vi "Make Graph.vi"(10 "SciData":dbl[][](array[numeric]), 11 "X-Data":dbl[](array[numeric])) -> (3 "All Counts 2":cluster{"X-Data":dbl[], "SciData":dbl[]}[](graph))   [LabVIEW 2025]
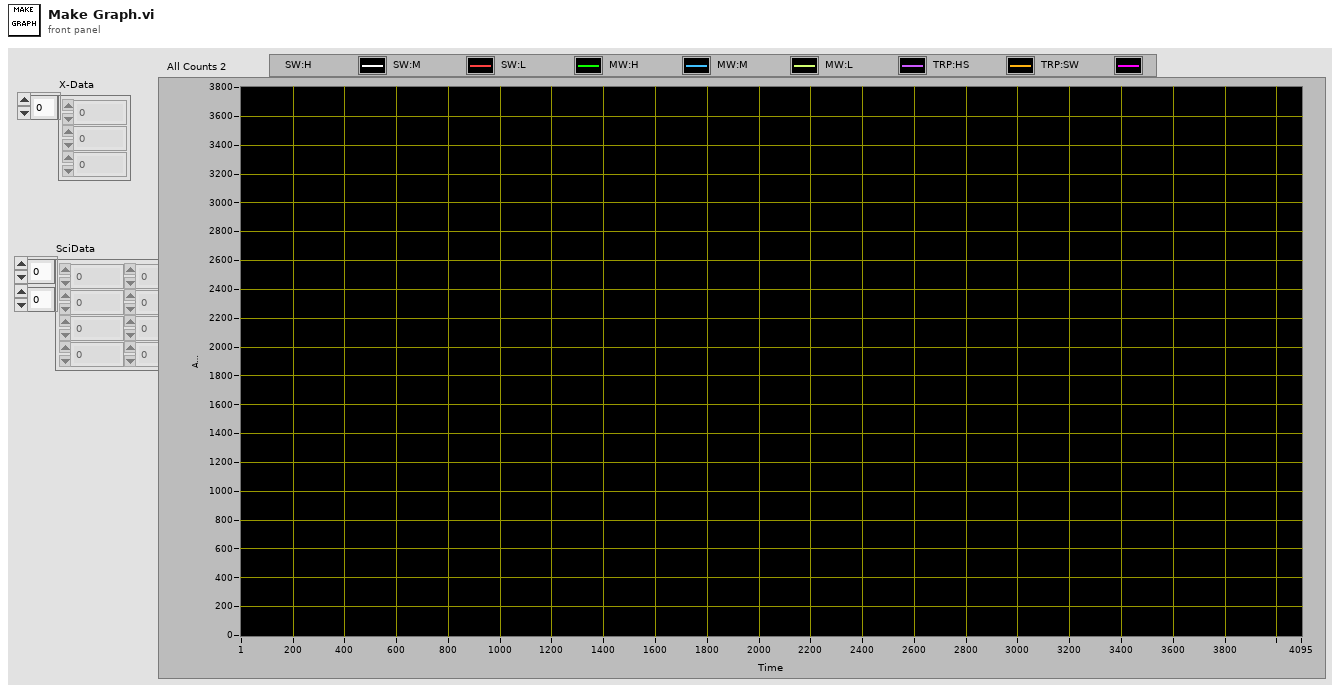
[diagram p1: front panel]
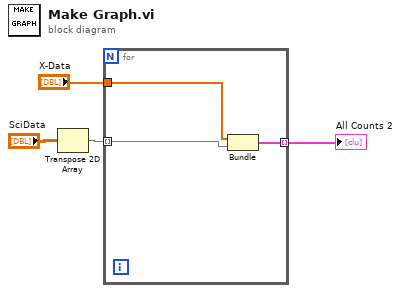
[diagram p0: block diagram]
diagram:
  n1 = Transpose 2D Array(2D array="SciData") -> (transposed array=w1:dbl[][])
  n2 = for {
    tunnel: w1 -> [w7] mode=indexing
    tunnel: "X-Data" -> [w6]
    tunnel: [w5] -> w2 mode=indexing
    n3 = Bundle("X-Data"=w6, w7) -> (w5:cluster{"X-Data":dbl[], dbl[]})  [unwired: 1 in]
  }
  "All Counts 2" <- w2
